vi "传递引用.vi"() -> ()   [LabVIEW 2013]
uses:
  <vilib>/Platform/TimedLoop/XDataNode/timing_clust.ctl
  <vilib>/Platform/TimedLoop/XDataNode/nitl_modes.ctl
  <vilib>/Platform/TimedLoop/XDataNode/wakeup.ctl
  <vilib>/Platform/TimedLoop/XDataNode/XDataNode.xnode
  <vilib>/Platform/TimedLoop/XDataNode/XDNodeRunTimeDep.lvlib
panel:
  in  "停止":bool
  out "数据值":dbl[](array[numeric])
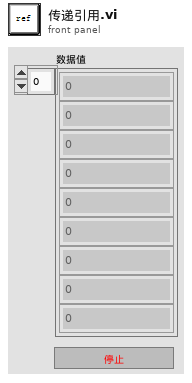
[diagram p1: front panel]
types:
  T1 = typedef "XDNodeRunTimeDep.lvlib/timing_clust.ctl" = cluster{"Expected End [f-1]":u64, "Actual End [f-1]":u64, "Finished Late? [f-1]":bool, "Expected End [i-1]":u64, "Actual End [i-1]":u64, "Finished Late? [i-1]":bool, "Expected Start [i]":u64, "Actual Start [i]":u64, "Expected Start [f]":u64, "Actual Start [f]":u64, "Source Name":string, "Structure Name":string, "Period":i64, "Deadline":i64, "Offset":i64, "Start":i64, "Priority":i32, "Timeout":i32, "Mode":T2, "Wakeup Reason":T3, "Error":errorcluster, "Source Type":string, "Secondary Source Type":string, "Global End Time":u64, "Global Start Time":u64, "Frame Duration":u64, "Iteration Duration":u64, "Assigned CPU":i32, "I/O Scan Engine Mode":u32}
  T2 = typedef "XDNodeRunTimeDep.lvlib/nitl_modes.ctl" = enum32{"No Change", "Process missed periods, maintain original phase", "Discard missed periods, maintain original phase", "Process missed periods, ignore original phase", "Discard missed periods, ignore original phase"}
  T3 = typedef "XDNodeRunTimeDep.lvlib/wakeup.ctl" = enum32{"Normal", "Aborted", "Asynchronous wakeup", "Timing source error", "Timed loop error", "Timeout"}
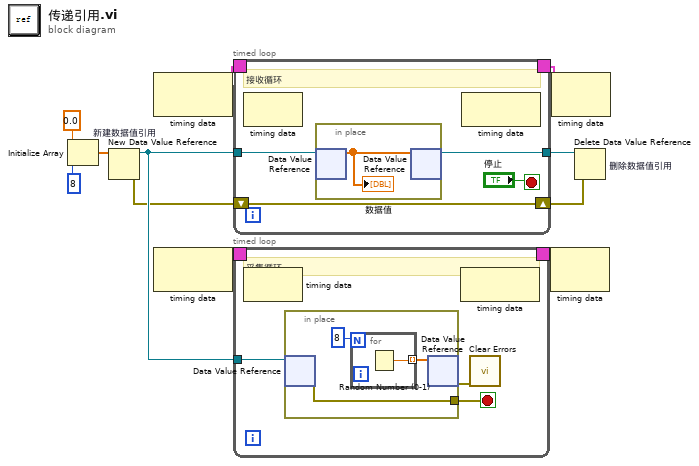
[diagram p0: block diagram]
diagram:
  n1 = Initialize Array(0.0 ("元素"), 8 ("维数大小")) -> (w7:dbl[])
  n2 = New Data Value Reference "新建数据值引用"(data value=w7) -> (data value reference=w4:refnum<data-value>, error out=w3:errorcluster)  [unwired: 1 in]
  n3 = node-c288() -> (w6:T1)  [unwired: 1 in]
  n4 = node-c288() -> (w11:T1)  [unwired: 1 in]
  n5 = timed-loop {
    timing: w6 -> [_]
    timing-out: [_] -> w5
    tunnel: w4 -> [w15]
    shift-right: [w13] -> w2
    shift-left: w3 -> [w13]
    tunnel: [w12] -> w1
    stop <- "停止" stop-if-true
    # "接收循环"
    n6 = node-c288() -> ()  [unwired: 1 in, 1 out]
    n7 = in-place {
      n8 = in-place-dvr #1(w15) -> (w16:dbl[])  [unwired: 1 out]
      "数据值" <- w16
      n9 = in-place-dvr #1(w16) -> (w12:refnum<data-value>)  [unwired: 1 out]
    }
    n10 = node-c288() -> ()  [unwired: 1 in, 1 out]
  }
  n11 = timed-loop {
    timing: w11 -> [_]
    timing-out: [_] -> w10
    tunnel: w4 -> [w21]
    stop <- w20 stop-if-true
    # "采集循环"
    n12 = node-c288() -> ()  [unwired: 1 in, 1 out]
    n13 = in-place {
      in-place-border: [w22] -> w20
      n14 = in-place-dvr #2(w21) -> (w22:errorcluster)  [unwired: 1 out]
      n15 = for {
        N: 8 -> [_]
        tunnel: [w25] -> w23 mode=indexing
        n16 = Random Number (0-1)() -> (number: 0 to 1=w25:dbl)
      }
      n17 = in-place-dvr #2(w23) -> (w19:errorcluster)  [unwired: 1 out]
    }
    n18 = node-c288() -> ()  [unwired: 1 in, 1 out]
    n19 = call <vilib>:"Clear Errors.vi"("error in (no error)"=w19) -> ()  [unwired: 6 in, 1 out]
  }
  n20 = node-c288(w10) -> ()  [unwired: 1 out]
  n21 = node-c288(w5) -> ()  [unwired: 1 out]
  n22 = Delete Data Value Reference "删除数据值引用"(data value reference=w1, error in=w2) -> ()  [unwired: 2 out]
